vi "SetChamber.vi"(3 "Code":i32(ring) items=["Seal", "PurgeAndSeal", "VentAndSeal", "PumpContinuous", "VentContinuous", "HighVacuum"], 4 "error in (no error)":errorcluster, 5 "Instrument Ref In":refnum<k24>) -> (0 "SetChamber Error":i32, 1 "error out":errorcluster, 2 "Instrument Ref Out":refnum<k24>)   [LabVIEW 2019]
uses:
  QDInstrument.dll
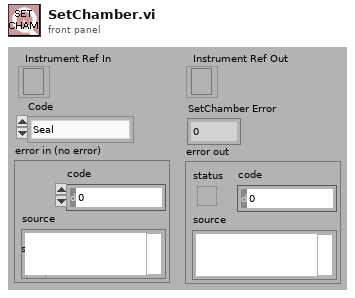
[diagram p1: front panel]
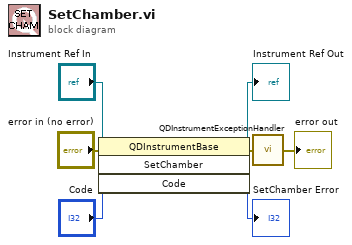
[diagram p0: block diagram]
diagram:
  n1 = invoke class="QDInstrumentBase" method="SetChamber"(reference="Instrument Ref In", error in="error in (no error)", "Code"="Code") -> (reference out=→"Instrument Ref Out":refnum<k24>, error out=w2:errorcluster, "SetChamber"=→"SetChamber Error":i32)  [unwired: 1 in, 1 out]
  n2 = call "QDInstrumentExceptionHandler.vi"("Error in"=w2) -> ("Error out"=→"error out":errorcluster)
